vi "Two Button Screen.vi"() -> ()   [LabVIEW 2011]
uses:
  op_typdef.ctl
panel:
  in  "Ignore Button":bool
  in  "Message":string
  out "Op Out":T1
  in  "OK Button":bool
  in  "Stop Button":bool
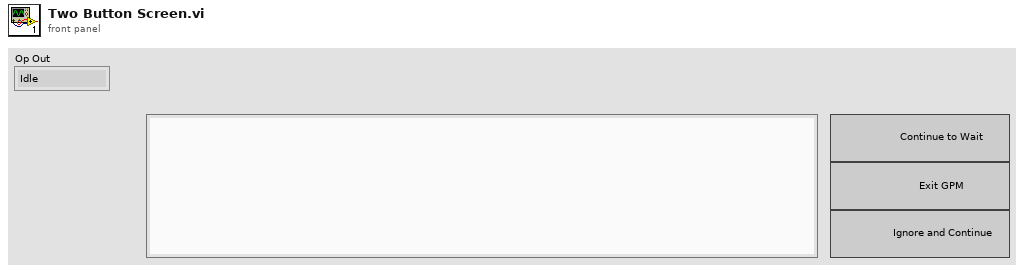
[diagram p1: front panel]
types:
  T1 = typedef "op_typdef.ctl" = enum16{"Idle", "Continue to Wait", "Exit", "Ignore and Continue"}
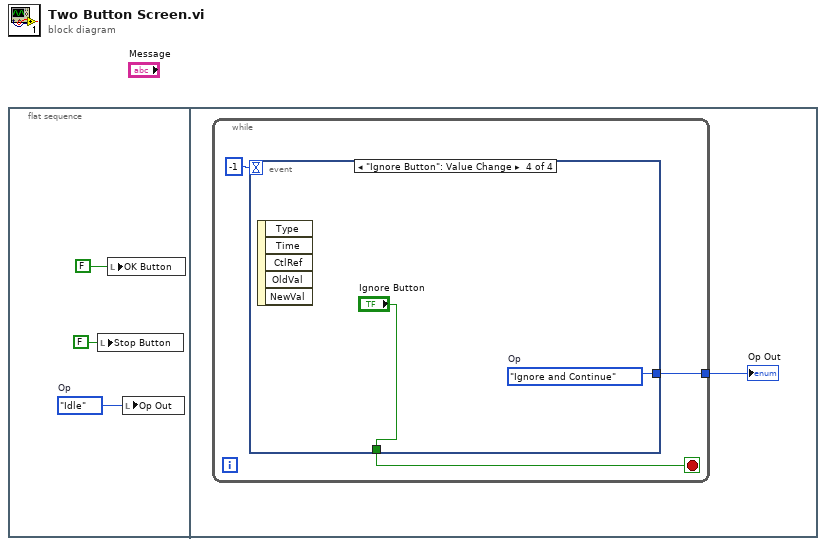
[diagram p0: block diagram]
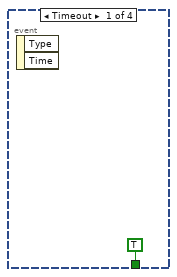
[diagram p2: hidden frame]
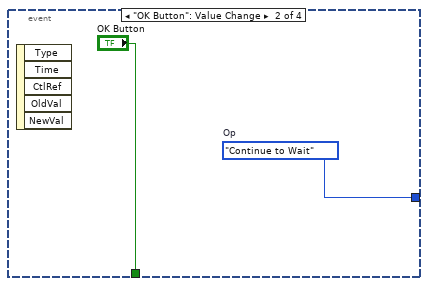
[diagram p3: hidden frame]
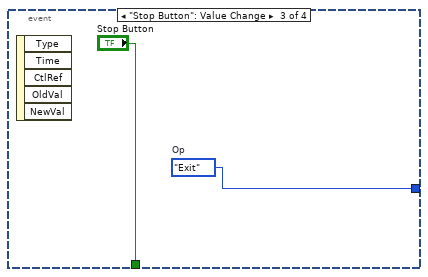
[diagram p4: hidden frame]
diagram:
  n1 = flat-sequence {
    frame #0 {
      w1 = op_typdef."Idle"  # Op
      n2 = local write "Stop Button"(FALSE ("Stop Button")) -> ()
      n3 = local write "OK Button"(FALSE ("OK Button")) -> ()
      n4 = local write "Op Out"(w1) -> ()
    }
    frame #1 {
      n5 = while {
        tunnel: [w6] -> w4
        stop <- w5 stop-if-true
        n6 = event shown="[3] \"Ignore Button\": Value Change" {
          selector: _ -> [_ _ _ _]
          dyn-events: _ -> [_ _ _ _]
          timeout: -1 ("Numeric") -> [_ _ _ _]
          tunnel: [_ w10 w12 w13] -> w6
          tunnel: [TRUE ("Stop Button") "OK Button" "Stop Button" "Ignore Button"] -> w5
          event Timeout {
            n7 = event-data() -> ()  [unwired: 1 in, 2 out]
          }
          event "OK Button": Value Change {
            w10 = op_typdef."Continue to Wait"  # Op
            n8 = event-data() -> ()  [unwired: 1 in, 5 out]
          }
          event "Stop Button": Value Change {
            w12 = op_typdef."Exit"  # Op
            n9 = event-data() -> ()  [unwired: 1 in, 5 out]
          }
          event "Ignore Button": Value Change {
            w13 = op_typdef."Ignore and Continue"  # Op
            n10 = event-data() -> ()  [unwired: 1 in, 5 out]
          }
        }
      }
      "Op Out" <- w4
    }
  }
